vi "rvc Homogeneous to Euler.vi"(8 "error in (no error)":errorcluster, 11 "T":dbl[][](array[numeric])) -> (0 "Error Out":errorcluster, 1 "y":dbl, 2 "x":dbl, 3 "Array":dbl[](array[numeric]), 4 "z":dbl)   [LabVIEW 2014]
uses:
  <vilib>/Utility/error.llb/Error Cluster From Error Code.vi
  <vilib>/ErrorRing/Error Ring.xnode
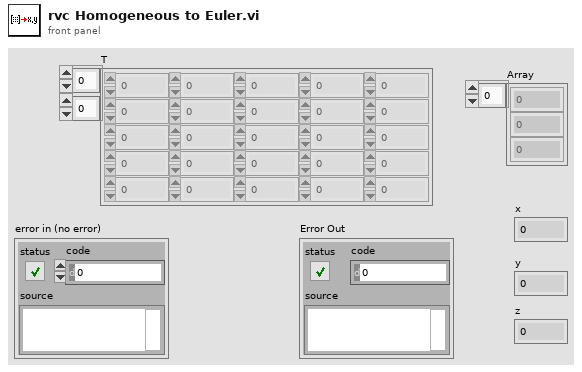
[diagram p1: front panel]
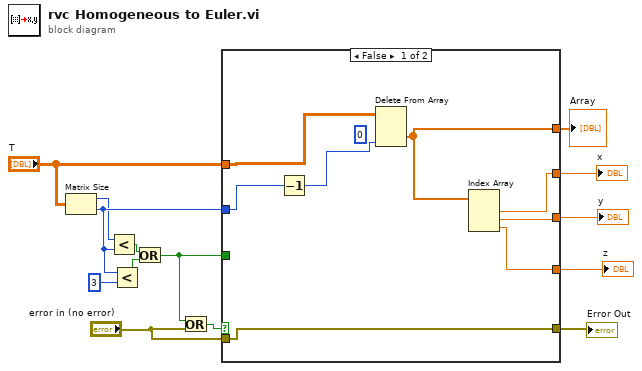
[diagram p0: block diagram]
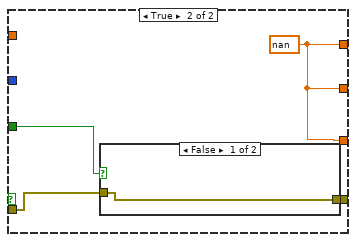
[diagram p2: hidden frame]
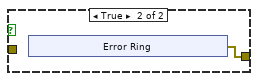
[diagram p3: hidden frame]
diagram:
  n1 = Matrix Size(0:"T") -> (1:w2:i32, 2:w8:i32)
  n2 = Less?(x=w2, y=w8) -> (x < y?=w10:bool)
  n3 = Less?(x=w8, y=3) -> (x < y?=w9:bool)
  n4 = Or(x=w10, y=w9) -> (x .or. y?=w5:bool)
  n5 = Or(x=w5, y="error in (no error)") -> (x .or. y?=w7:bool)
  n6 = case shown="False" w7 {
    tunnel: [w21 w24] -> w14
    tunnel: "T" -> [w20 _]
    tunnel: w8 -> [w22 _]
    tunnel: [w17 w23] -> w12
    tunnel: [w16 w23] -> w11
    tunnel: "error in (no error)" -> [w21 w25]
    tunnel: w5 -> [_ w26]
    tunnel: [w18 _] -> w4
    tunnel: [w15 w23] -> w3
    frame False {
      (unwired) 0 ("index (row)")
      n7 = Decrement(x=w22) -> (x-1=w19:i32)
      n8 = Delete From Array(array=w20, index (col)=w19) -> (deleted portion=w18:dbl[])  [unwired: 2 in, 1 out]
      n9 = Index Array(array=w18) -> (element #1=w17:dbl, element #2=w16:dbl, element #3=w15:dbl)  [unwired: 3 in]
    }
    frame True {
      w23 = nan ("x")
      n10 = case shown="False" w26 {
        tunnel: w25 -> [w27 _]
        tunnel: [w27 w28] -> w24
        frame False {
        }
        frame True {
          n11 = xnode "Error Ring"() -> ("error out"=w28:errorcluster)
        }
      }
    }
  }
  "x" <- w12
  "y" <- w11
  "Error Out" <- w14
  "Array" <- w4
  "z" <- w3
